vi "outFrame.vi"(6 "Sensor Array":bool[](array[boolean]), 7 "Select Macro Function":T1(radio), 8 "error in (no error)":errorcluster, 9 "On/Off Data":bool, 10 "Write Data (HEX)":string, 11 "Cluster in":refnum<vi>) -> (0 "error out":errorcluster, 1 "H2F Frame":string)   [LabVIEW 2018]
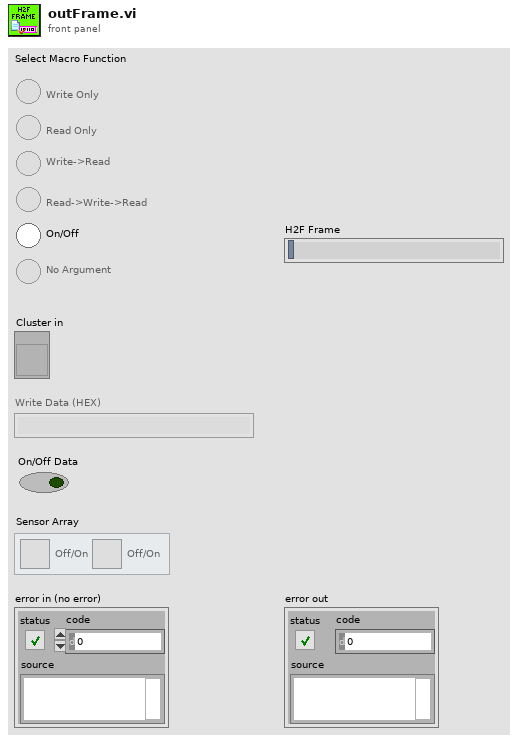
[diagram p1: front panel]
types:
  T1 = enum32{"No Selection", "WRITE", "READ", "WRITE -> READ", "READ -> WRITE -> READ", "ON/OFF", "NO ARGS"}
  T2 = typedef "dictCluster.ctl" = cluster{"D_ID":string, "D_ID_NAME":string, "D_TYPE":string, "WRITE":bool, "READ":bool, "W_R":bool, "R_W_R":bool, "D_VOID":bool, "ON_OFF":bool, "DATA_SIZE":u8}
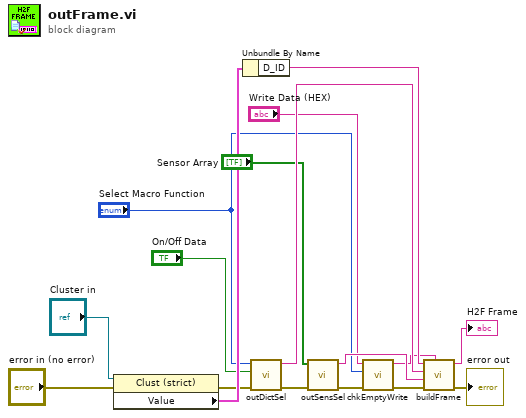
[diagram p0: block diagram]
diagram:
  n1 = property on="Property Node" class="Clust (strict)"(reference="Cluster in", error in="error in (no error)") -> (error out=w3:errorcluster, "Value"=w14:T2)  [unwired: 1 out]
  n2 = Unbundle By Name(w14) -> ("D_ID"=w15:string)
  n3 = call "outDictSel.vi"("error in (no error)"=w3, "On/Off Data"="On/Off Data", "Select Macro Function"="Select Macro Function") -> ("error out"=w2:errorcluster, "Dictionary Selector"=w11:string)  [unwired: 7 in]
  n4 = call "outSensSel.vi"("error in (no error)"=w2, "Sensor Array"="Sensor Array") -> ("error out"=w1:errorcluster, "Sensor Selector"=w12:string)  [unwired: 8 in]
  n5 = call "chkEmptyWrite.vi"("error in (no error)"=w1, "Select Macro Function"="Select Macro Function", "Write Data (HEX)"="Write Data (HEX)") -> ("error out"=w9:errorcluster, "Write Data Out"=w10:string)  [unwired: 7 in]
  n6 = call "buildFrame.vi"("Data"=w10, "error in"=w9, "Sensor Selector"=w12, "Dictionary Selector"=w11, "Dictionary ID"=w15) -> ("error out"=→"error out":errorcluster, "H2F Frame"=→"H2F Frame":string)  [unwired: 3 in, 2 out]
